vi "bapsf_motion.vi"(4 "error in":errorcluster, 6 "Request data":variant, 7 "Request":string) -> (0 "error out":errorcluster, 2 "Response data":variant)   [LabVIEW 2022 SP3]
uses:
  typedefs/Device-specific request defs.ctl
panel:
  in  "py interface file":path
  in  "Python session":refnum<k35>
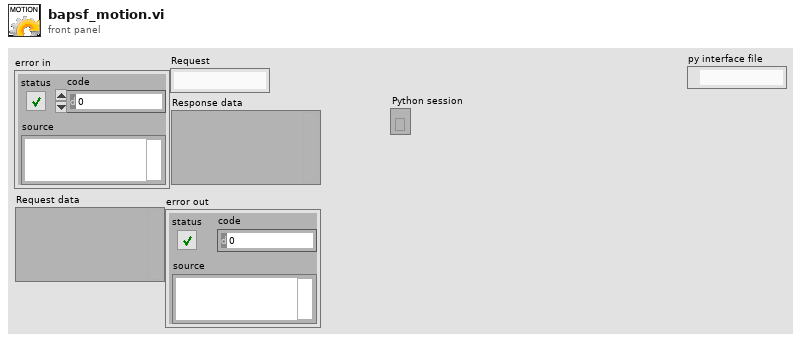
[diagram p1: front panel]
types:
  T1 = typedef "Device-specific request defs.ctl" = cluster{"Request":string, "Key-value types":cluster{"Key":string, "Value type":enum16{"<string>", "<int>"}}[]}[]
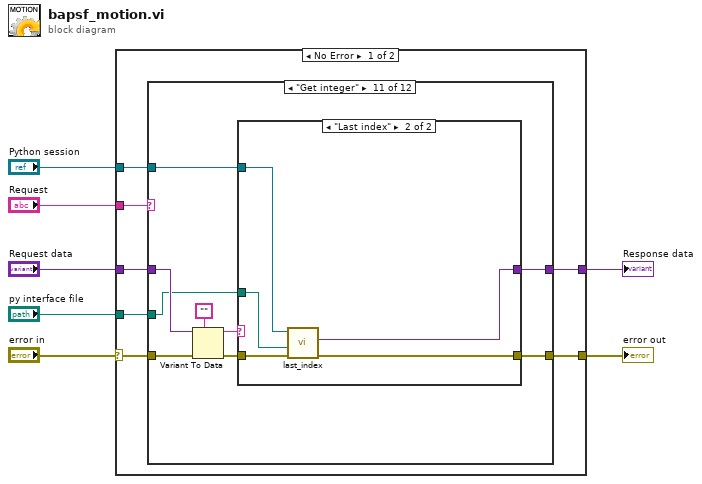
[diagram p0: block diagram]
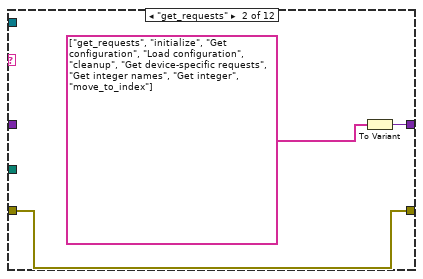
[diagram p3: hidden frame]
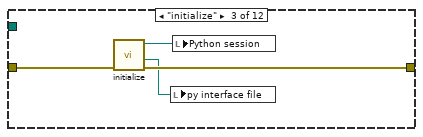
[diagram p4: hidden frame]
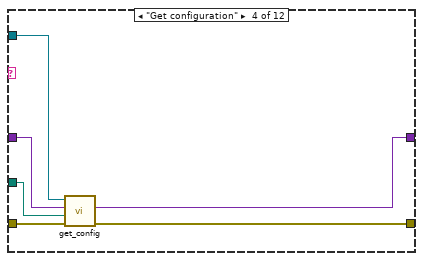
[diagram p5: hidden frame]
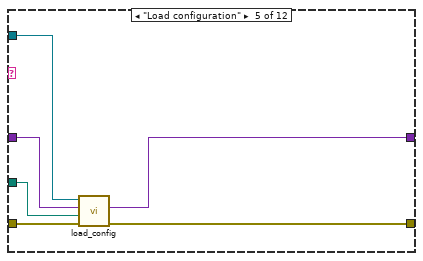
[diagram p6: hidden frame]
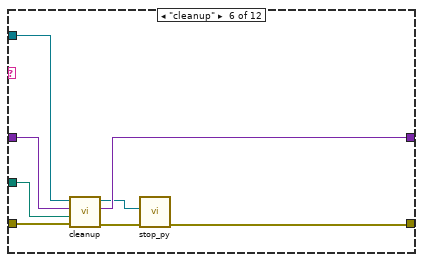
[diagram p7: hidden frame]
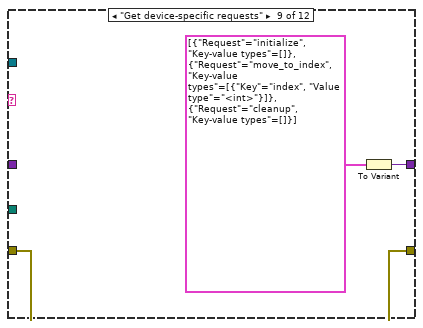
[diagram p10: hidden frame]
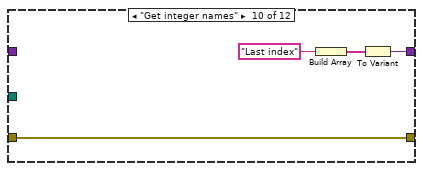
[diagram p11: hidden frame]
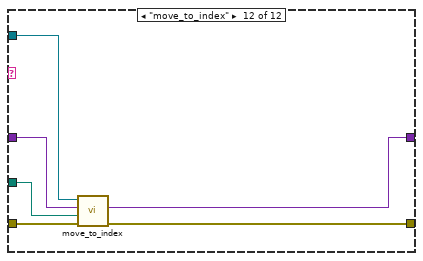
[diagram p13: hidden frame]
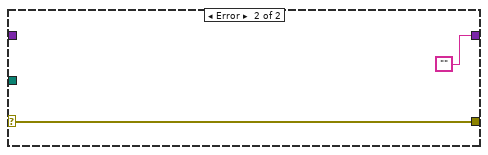
[diagram p14: hidden frame]
diagram:
  n1 = case shown="No Error" "error in" {
    selector: "error in" -> [w13 w77]
    tunnel: [w11 w77] -> w6
    tunnel: "Request" -> [w14 _]
    tunnel: "Request data" -> [w12 _]
    tunnel: [w10 ""] -> w3
    tunnel: "Python session" -> [w9 _]
    tunnel: "py interface file" -> [w8 _]
    frame No Error {
      n2 = case shown="\"Get integer\"" w14 {
        tunnel: w13 -> [w16 w19 w22 w29 w35 w43 w45 w47 w48 w54 w63 w75]
        tunnel: w12 -> [w15 _ _ w28 w33 w41 w44 w46 _ _ w62 w73]
        tunnel: [w16 w19 w23 w27 w31 w37 w45 w47 w48 w54 w57 w71] -> w11
        tunnel: [w15 w18 _ w26 w30 w39 w44 w46 w49 w51 w55 w70] -> w10
        tunnel: w9 -> [_ _ _ w25 w32 w40 _ _ _ _ w58 w72]
        tunnel: w8 -> [_ _ _ w24 w34 w42 _ _ _ _ w56 w74]
        frame "", Default {
        }
        frame "get_requests" {
          n3 = To Variant(anything=string[] ["get_requests", "initialize", "Get configuration", "Load configuration", "cleanup", "Get device-specific requests", "Get integer names", "Get integer", "move_to_index"]) -> (Variant=w18:variant)
        }
        frame "initialize" {
          n4 = call "initialize.vi"("error in (no error)"=w22) -> ("error out"=w23:errorcluster, "py interface file"=w21:path, "Python session out"=w20:refnum<k35>)  [unwired: 4 in]
          n5 = local write "py interface file"(w21) -> ()
          n6 = local write "Python session"(w20) -> ()
        }
        frame "Get configuration" {
          n7 = call "get_config.vi"("error in (no error)"=w29, "py interface file"=w24, "Request data"=w28, "Python session in"=w25) -> ("error out"=w27:errorcluster, "Response data"=w26:variant)  [unwired: 1 in, 1 out]
        }
        frame "Load configuration" {
          n8 = call "load_config.vi"("error in (no error)"=w35, "py interface file"=w34, "Request data"=w33, "Python session in"=w32) -> ("error out"=w31:errorcluster, "Response data"=w30:variant)  [unwired: 1 in, 1 out]
        }
        frame "cleanup" {
          n9 = call "cleanup.vi"("error in (no error)"=w43, "py interface file"=w42, "Request data"=w41, "Python session in"=w40) -> ("error out"=w38:errorcluster, "Response data"=w39:variant, "Python session out"=w36:refnum<k35>)  [unwired: 1 in]
          n10 = call "stop_py.vi"("error in"=w38, "Python session"=w36) -> ("error out"=w37:errorcluster)  [unwired: 5 in]
        }
        frame "Configure" {
        }
        frame "Get run-time state" {
        }
        frame "Get device-specific requests" {
          n11 = To Variant(anything=T1 [{"Request"="initialize", "Key-value types"=[]}, {"Request"="move_to_index", "Key-value types"=[{"Key"="index", "Value type"=enum."<int>"}]}, {"Request"="cleanup", "Key-value types"=[]}] ("Device-specific request defs")) -> (Variant=w49:variant)
        }
        frame "Get integer names" {
          n12 = Build Array("Last index") -> (w53:string[])
          n13 = To Variant(anything=w53) -> (Variant=w51:variant)
        }
        frame "Get integer" {
          n14 = Variant To Data(error in=w63, type="", Variant=w62) -> (data=w60:string, error out=w59:errorcluster)
          n15 = case shown="\"Last index\"" w60 {
            tunnel: w59 -> [w64 w69]
            tunnel: w58 -> [_ w67]
            tunnel: [w64 w66] -> w57
            tunnel: w56 -> [_ w68]
            tunnel: [_ w65] -> w55
            frame "", Default {
            }
            frame "Last index" {
              n16 = call "last_index.vi"("error in (no error)"=w69, "py interface file"=w68, "Python session in"=w67) -> ("error out"=w66:errorcluster, "Response data"=w65:variant)  [unwired: 2 in, 1 out]
            }
          }
        }
        frame "move_to_index" {
          n17 = call "move_to_index.vi"("error in (no error)"=w75, "py interface file"=w74, "Request data"=w73, "Python session in"=w72) -> ("error out"=w71:errorcluster, "Response data"=w70:variant)  [unwired: 1 in, 1 out]
        }
      }
    }
    frame Error {
    }
  }
  "Response data" <- w3
  "error out" <- w6
